vi "CRYImp wiz decide action.vi"(7 "Iteration":i32, 10 "New controls":T1, 11 "Old controls":T1) -> (3 "Frames to run":string[](array[string]))   [LabVIEW 2013]
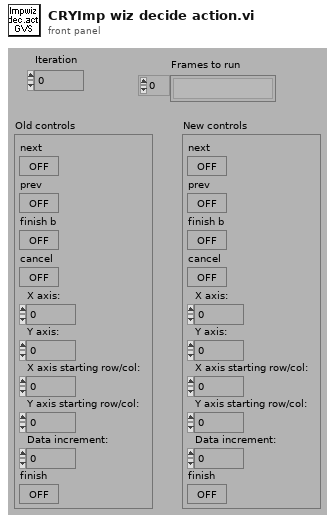
[diagram p1: front panel]
types:
  T1 = cluster{"next":bool, "prev":bool, "finish b":bool, "cancel":bool, "X axis:":i32, "Y axis:":i32, "X axis starting row/col:":i32, "Y axis starting row/col:":i32, "Data increment:":i32, "finish":bool}
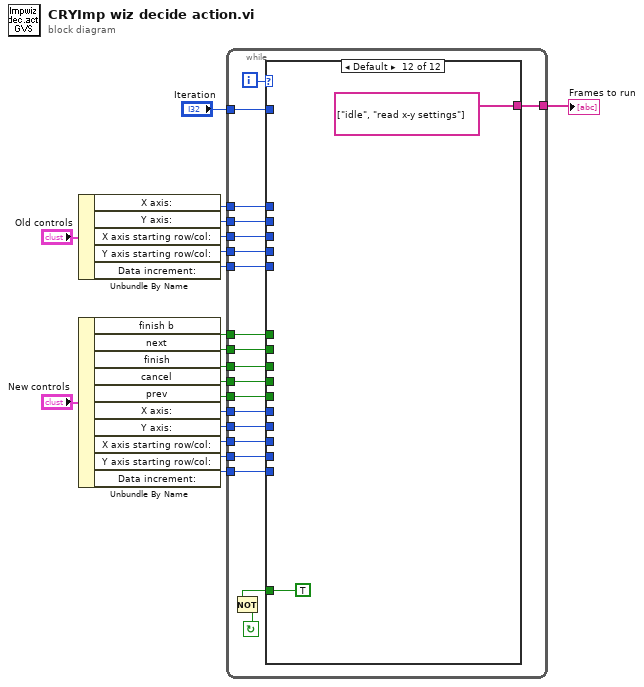
[diagram p0: block diagram]
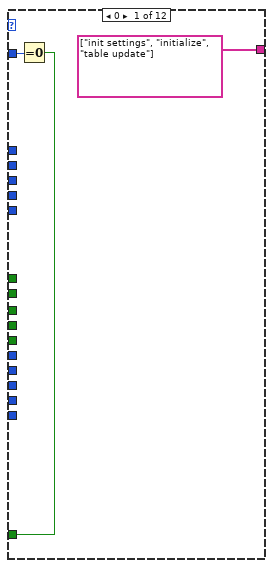
[diagram p2: hidden frame]
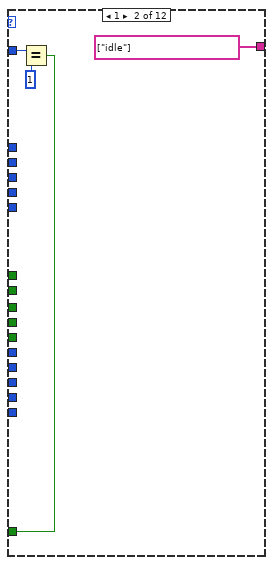
[diagram p3: hidden frame]
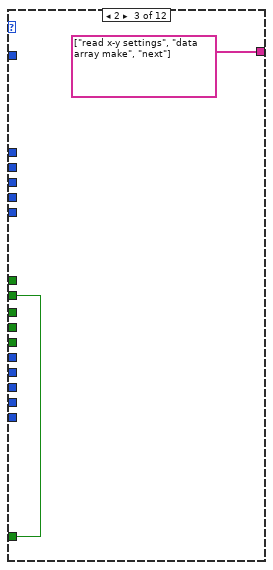
[diagram p4: hidden frame]
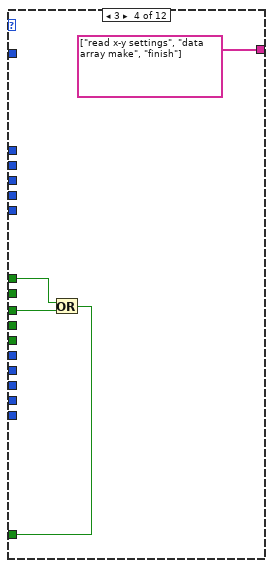
[diagram p5: hidden frame]
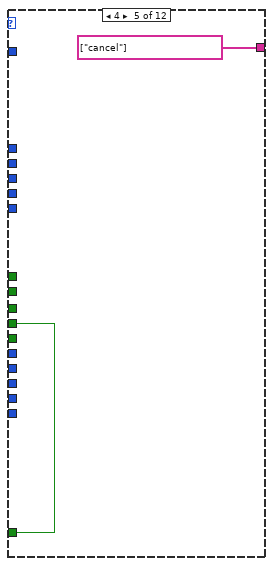
[diagram p6: hidden frame]
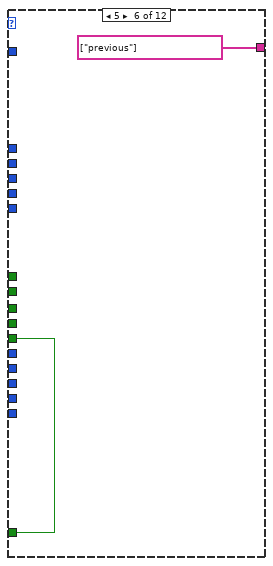
[diagram p7: hidden frame]
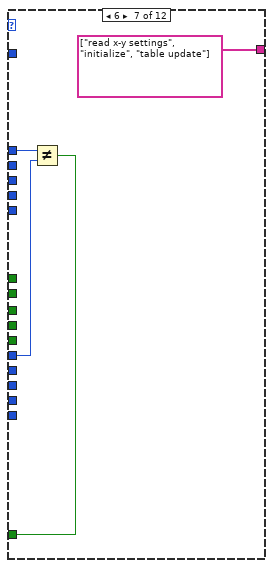
[diagram p8: hidden frame]
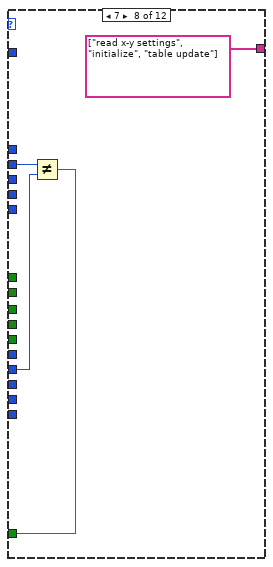
[diagram p9: hidden frame]
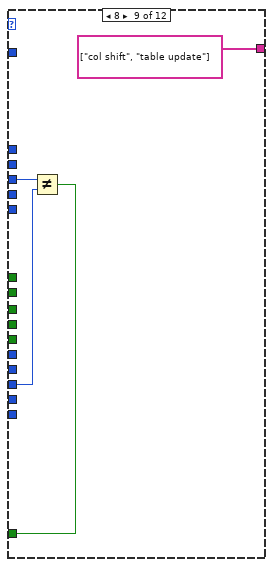
[diagram p10: hidden frame]
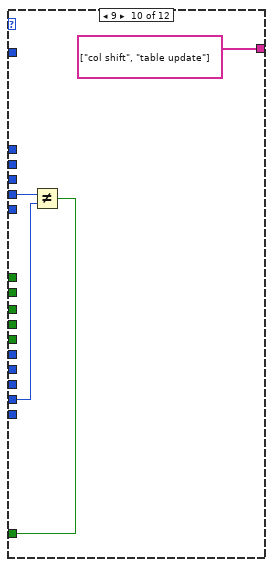
[diagram p11: hidden frame]
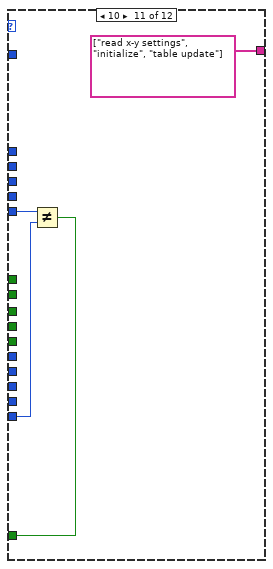
[diagram p12: hidden frame]
diagram:
  n1 = Unbundle By Name("Old controls") -> ("X axis:"=w11:i32, "Y axis:"=w9:i32, "X axis starting row/col:"=w7:i32, "Y axis starting row/col:"=w6:i32, "Data increment:"=w5:i32)
  n2 = Unbundle By Name("New controls") -> ("finish b"=w1:bool, "next"=w16:bool, "finish"=w15:bool, "cancel"=w14:bool, "prev"=w12:bool, "X axis:"=w10:i32, "Y axis:"=w8:i32, "X axis starting row/col:"=w4:i32, "Y axis starting row/col:"=w3:i32, "Data increment:"=w2:i32)
  n3 = while {
    tunnel: w1 -> [w20]
    tunnel: w2 -> [w21]
    tunnel: w3 -> [w22]
    tunnel: w4 -> [w23]
    tunnel: w5 -> [w24]
    tunnel: w6 -> [w25]
    tunnel: w7 -> [w26]
    tunnel: w8 -> [w27]
    tunnel: w9 -> [w28]
    tunnel: w10 -> [w29]
    tunnel: w11 -> [w30]
    tunnel: w12 -> [w31]
    tunnel: [w32] -> w13
    tunnel: w14 -> [w35]
    tunnel: w15 -> [w36]
    tunnel: w16 -> [w37]
    tunnel: "Iteration" -> [w38]
    i -> [w39]
    stop <- w33 continue-if-true
    n4 = case shown="Default" w39 {
      tunnel: w38 -> [w42 w44 _ _ _ _ _ _ _ _ _ _]
      tunnel: w37 -> [_ _ w48 _ _ _ _ _ _ _ _ _]
      tunnel: w36 -> [_ _ _ w51 _ _ _ _ _ _ _ _]
      tunnel: w35 -> [_ _ _ _ w53 _ _ _ _ _ _ _]
      tunnel: [w41 w43 w48 w49 w53 w55 w59 w64 w67 w71 w76 TRUE] -> w34
      tunnel: [string[] ["init settings", "initialize", "table update"] string[] ["idle"] string[] ["read x-y settings", "data array make", "next"] string[] ["read x-y settings", "data array make", "finish"] string[] ["cancel"] string[] ["previous"] string[] ["read x-y settings", "initialize", "table update"] string[] ["read x-y settings", "initialize", "table update"] string[] ["col shift", "table update"] string[] ["col shift", "table update"] string[] ["read x-y settings", "initialize", "table update"] string[] ["idle", "read x-y settings"]] -> w32
      tunnel: w31 -> [_ _ _ _ _ w55 _ _ _ _ _ _]
      tunnel: w30 -> [_ _ _ _ _ _ w58 _ _ _ _ _]
      tunnel: w29 -> [_ _ _ _ _ _ w57 _ _ _ _ _]
      tunnel: w28 -> [_ _ _ _ _ _ _ w63 _ _ _ _]
      tunnel: w27 -> [_ _ _ _ _ _ _ w62 _ _ _ _]
      tunnel: w26 -> [_ _ _ _ _ _ _ _ w66 _ _ _]
      tunnel: w25 -> [_ _ _ _ _ _ _ _ _ w70 _ _]
      tunnel: w24 -> [_ _ _ _ _ _ _ _ _ _ w75 _]
      tunnel: w23 -> [_ _ _ _ _ _ _ _ w65 _ _ _]
      tunnel: w22 -> [_ _ _ _ _ _ _ _ _ w69 _ _]
      tunnel: w21 -> [_ _ _ _ _ _ _ _ _ _ w74 _]
      tunnel: w20 -> [_ _ _ w50 _ _ _ _ _ _ _ _]
      frame 0 {
        n5 = Equal To 0?(x=w42) -> (x = 0?=w41:bool)
      }
      frame 1 {
        n6 = Equal?(x=w44, y=1) -> (x = y?=w43:bool)
      }
      frame 2 {
      }
      frame 3 {
        n7 = Or(x=w50, y=w51) -> (x .or. y?=w49:bool)
      }
      frame 4 {
      }
      frame 5 {
      }
      frame 6 {
        n8 = Not Equal?(x=w58, y=w57) -> (x != y?=w59:bool)
      }
      frame 7 {
        n9 = Not Equal?(x=w63, y=w62) -> (x != y?=w64:bool)
      }
      frame 8 {
        n10 = Not Equal?(x=w66, y=w65) -> (x != y?=w67:bool)
      }
      frame 9 {
        n11 = Not Equal?(x=w70, y=w69) -> (x != y?=w71:bool)
      }
      frame 10 {
        n12 = Not Equal?(x=w75, y=w74) -> (x != y?=w76:bool)
      }
      frame Default {
      }
    }
    n13 = Not(x=w34) -> (.not. x?=w33:bool)
  }
  "Frames to run" <- w13
